vi "Cleanup Compiled Settings.vi"(11 "Output Sequencer in":refnum<class "Output Sequencer.lvclass">) -> (0 "error out":errorcluster, 3 "Output Sequencer out":refnum<class "Output Sequencer.lvclass">)   [LabVIEW 2024, in "Output Sequencer.lvlib" / "Output Sequencer.lvclass"]
uses:
  Output Sequencer.lvclass
  Types/Compiled Settings.ctl
  Types/Expression Data.ctl
  <vilib>/LAVA/muParser/mupExpr/mupExpr.lvclass
  Types/Compiled Step.ctl
  Output Sequencer.lvclass/Output Sequencer.ctl
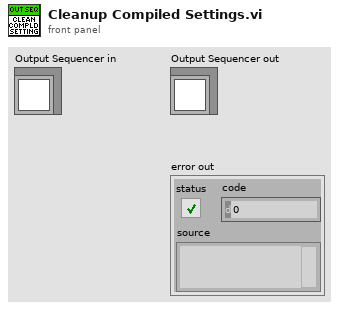
[diagram p1: front panel]
types:
  T1 = typedef "Output Sequencer.lvlib/Output Sequencer.lvclass/Compiled Settings.ctl" = cluster{"Start condition":T2, "Stop Condition":T2, "Compiled Steps":T3[]}
  T2 = typedef "Output Sequencer.lvlib/Output Sequencer.lvclass/Expression Data.ctl" = cluster{"Empty?":bool, "Expression":refnum<class "mupExpr.lvclass">, "Variable Names":string[]}
  T3 = typedef "Output Sequencer.lvlib/Output Sequencer.lvclass/Compiled Step.ctl" = cluster{"Precondition":T2, "Duration":dbl, "Mode":string, "Delay Between Values":dbl, "Analog Values":T2[], "Digital Values":T2[], "Postcondition":T2, "On True":string, "On False":string}
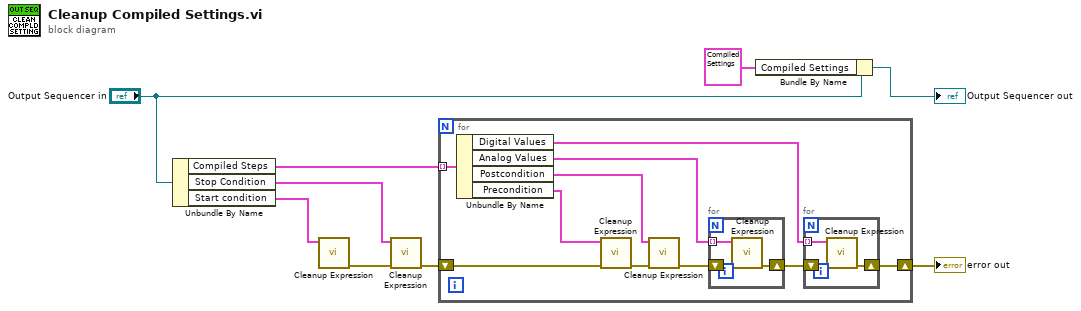
[diagram p0: block diagram]
diagram:
  n1 = Unbundle By Name("Output Sequencer in") -> ("Compiled Steps"=w9:T3[], "Stop Condition"=w4:T2, "Start condition"=w5:T2)
  n2 = call "Cleanup Expression.vi"("Expression Data"=w5) -> ("error out"=w3:errorcluster)  [unwired: 10 in]
  n3 = call "Cleanup Expression.vi"("error in (no error)"=w3, "Expression Data"=w4) -> ("error out"=w2:errorcluster)  [unwired: 9 in]
  n4 = for {
    tunnel: w9 -> [w19] mode=indexing
    shift-right: [w10] -> w1
    shift-left: w2 -> [w18]
    n5 = Unbundle By Name(w19) -> ("Digital Values"=w11:T2[], "Analog Values"=w13:T2[], "Postcondition"=w16:T2, "Precondition"=w17:T2)
    n6 = call "Cleanup Expression.vi"("error in (no error)"=w18, "Expression Data"=w17) -> ("error out"=w15:errorcluster)  [unwired: 9 in]
    n7 = call "Cleanup Expression.vi"("error in (no error)"=w15, "Expression Data"=w16) -> ("error out"=w14:errorcluster)  [unwired: 9 in]
    n8 = for {
      shift-right: [w24] -> w12
      shift-left: w14 -> [w25]
      tunnel: w13 -> [w23] mode=indexing
      n9 = call "Cleanup Expression.vi"("error in (no error)"=w25, "Expression Data"=w23) -> ("error out"=w24:errorcluster)  [unwired: 9 in]
    }
    n10 = for {
      shift-right: [w21] -> w10
      shift-left: w12 -> [w22]
      tunnel: w11 -> [w20] mode=indexing
      n11 = call "Cleanup Expression.vi"("error in (no error)"=w22, "Expression Data"=w20) -> ("error out"=w21:errorcluster)  [unwired: 9 in]
    }
  }
  "error out" <- w1
  n12 = Bundle By Name(cluster="Output Sequencer in", "Compiled Settings"=T1 {"Start condition"={"Empty?"=FALSE, "Expression"=refnum, "Variable Names"=[]}, "Stop Condition"={"Empty?"=FALSE, "Expression"=refnum, "Variable Names"=[]}, "Compiled Steps"=[]}) -> (→"Output Sequencer out":refnum<class "Output Sequencer.lvclass">)
